vi "ReduceFileSize_SingleFile.vi"(7 "Appendix":string="_r", 8 "error in (no error)":errorcluster, 11 "appended path":path) -> (0 "error out":errorcluster, 3 "appended path 2":path)   [LabVIEW 2015, in "EMG.lvclass"]
uses:
  EMG.lvclass
  <vilib>/Utility/file.llb/Read From Spreadsheet File (string).vi
  <vilib>/Utility/file.llb/Write To Spreadsheet File (string).vi
  CustomVIs/CustomVI.lvlib
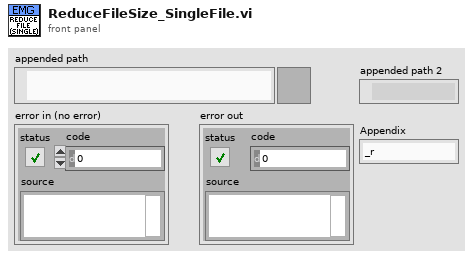
[diagram p1: front panel]
types:
  T1 = enum16{"open", "replace", "create", "open or create", "replace or create", "replace or create with confirmation"}
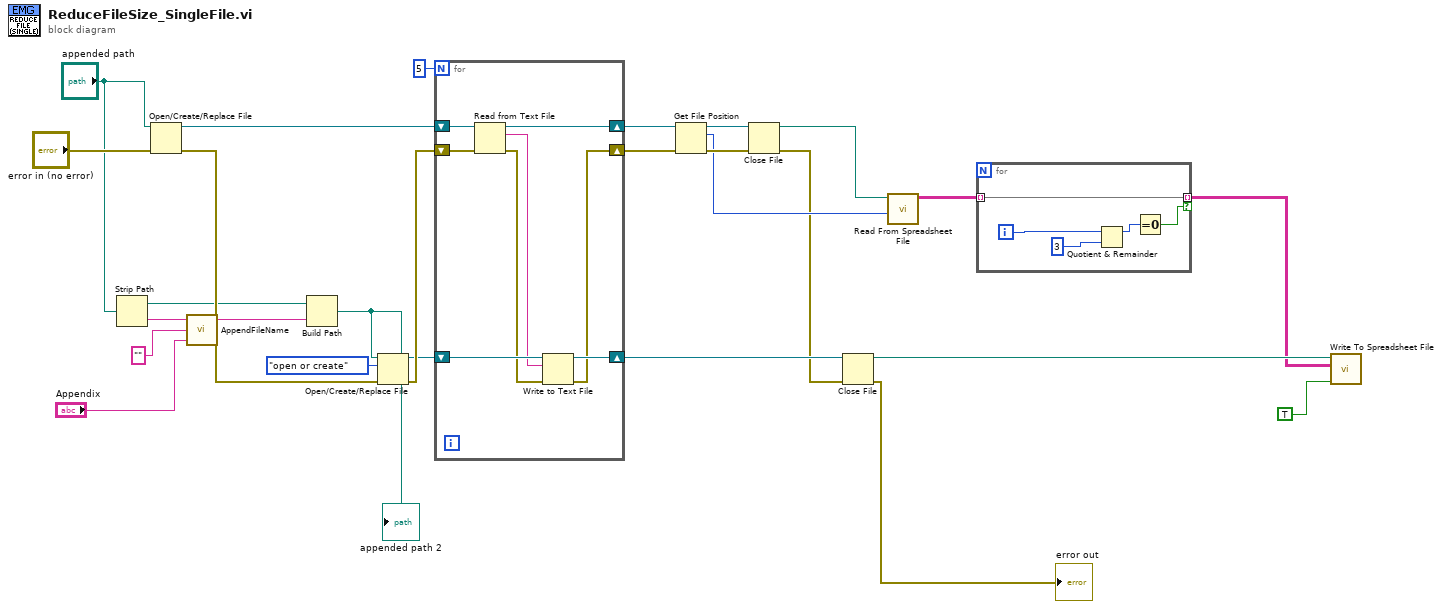
[diagram p0: block diagram]
diagram:
  n1 = Strip Path(path="appended path") -> (stripped path=w3:path, name=w4:string)
  n2 = Open/Create/Replace File(file path (use dialog)="appended path", error in="error in (no error)") -> (refnum out=w18:refnum<file>, error out=w23:errorcluster)  [unwired: 4 in, 1 out]
  n3 = call "AppendFileName.vi"("Appendix"="Appendix", "Sperator(_)"="", "Filename"=w4) -> ("New Filename"=w6:string)  [unwired: 2 in]
  n4 = Build Path(base path=w3, name or relative path=w6) -> (appended path=w20:path)
  "appended path 2" <- w20
  n5 = Open/Create/Replace File(file path (use dialog)=w20, error in=w23, operation (0:open)=T1."open or create") -> (refnum out=w22:refnum<file>, error out=w24:errorcluster)  [unwired: 3 in, 1 out]
  n6 = for {
    N: 5 -> [_]
    shift-right: [w33] -> w26
    shift-left: w18 -> [w35]
    shift-right: [w28] -> w27
    shift-left: w24 -> [w34]
    shift-right: [w31] -> w13
    shift-left: w22 -> [w32]
    n7 = Read from Text File(file (use dialog)=w35, error in=w34) -> (refnum out=w33:refnum<file>, text=w30:string, error out=w29:errorcluster)  [unwired: 2 in, 1 out]
    n8 = Write to Text File(file (use dialog)=w32, text=w30, error in=w29) -> (refnum out=w31:refnum<file>, error out=w28:errorcluster)  [unwired: 1 in, 1 out]
  }
  n9 = Get File Position(4:w27, 7:w26) -> (0:w16:errorcluster, 2:w14:i64, 3:w17:refnum<file>)
  n10 = Close File(refnum=w17, error in=w16) -> (path=w15:path, error out=w12:errorcluster)
  n11 = Close File(refnum=w13, error in=w12) -> (path=w11:path, error out=→"error out":errorcluster)
  n12 = call-poly <vilib>:"Read From Spreadsheet File.vi"("start of read offset (chars.:0)"=w14, "file path (dialog if empty)"=w15) -> ("all rows"=w8:string[][])  [unwired: 5 in, 4 out]
  n13 = for {
    tunnel: w8 -> [w38] mode=indexing
    tunnel: [w38] -> w7 mode=indexing if=w36
    i -> [w40]
    n14 = Quotient & Remainder(x=w40, y=3) -> (x-y*floor(x/y)=w37:i32)  [unwired: 1 out]
    n15 = Equal To 0?(x=w37) -> (x = 0?=w36:bool)
  }
  n16 = call-poly <vilib>:"Write To Spreadsheet File.vi"("append to file? (new file:F)"=TRUE, "2D data"=w7, "file path (dialog if empty)"=w11) -> ()  [unwired: 5 in, 1 out]
